vi "GetAllAxisPositions.vi"(8 "error in (no error)":errorcluster, 11 "Picomoto8742ControllerClass in":refnum<class "Picomoto8742ControllerClass.lvclass">) -> (0 "error out":errorcluster, 2 "AxisPositions":i32[](array[numeric]), 3 "Picomoto8742ControllerClass out":refnum<class "Picomoto8742ControllerClass.lvclass">)   [LabVIEW 2020, in "Picomoto8742ControllerClass.lvclass"]
doc: "Query all the axis positions from the physical device"
uses:
  Picomoto8742ControllerClass.lvclass
  Picomoto8742ControllerClass.lvclass/Picomoto8742ControllerClass.ctl
  PicoMotor8742Axis/Picomotor8742Axis.lvclass
panel:
  in  "milliseconds to wait":u32
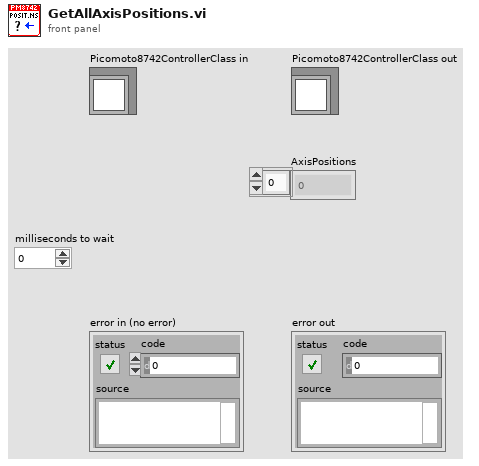
[diagram p1: front panel]
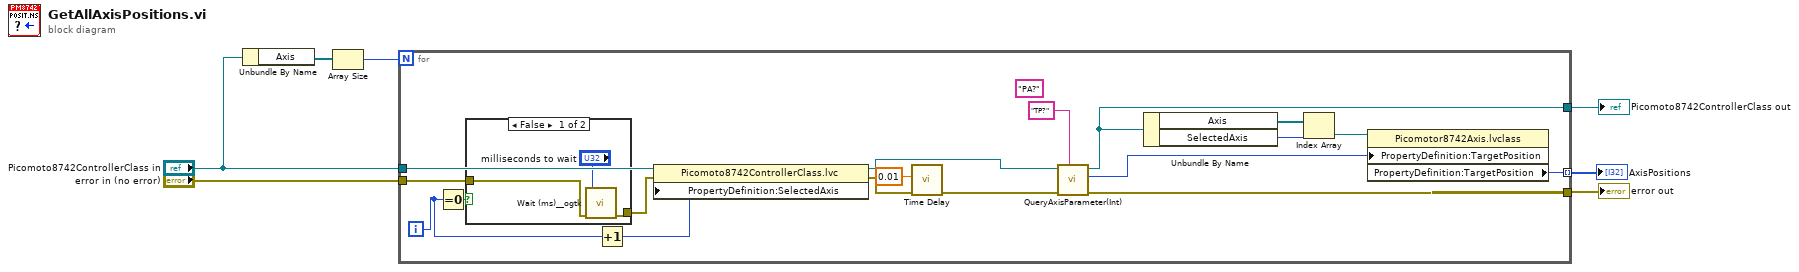
[diagram p0: block diagram]
diagram:
  n1 = Unbundle By Name("Picomoto8742ControllerClass in") -> ("Axis"=w4:refnum<class "Picomotor8742Axis.lvclass">[])
  n2 = Array Size(array=w4) -> (size(s)=w3:i32)
  n3 = for {
    N: w3 -> [_]
    tunnel: "Picomoto8742ControllerClass in" -> [w25]
    tunnel: [w19] -> w6
    tunnel: "error in (no error)" -> [w9]
    tunnel: [w14] -> w1 mode=indexing
    tunnel: [w13] -> w2
    i -> [w11]
    (unwired) "PA?" ("string")
    n4 = Equal To 0?(x=w11) -> (x = 0?=w10:bool)
    n5 = case shown="False" w10 {
      tunnel: w9 -> [w28 w29]
      tunnel: [w27 w29] -> w8
      frame False {
        n6 = call <userlib>:"Wait (ms)__ogtk.vi"("error in (no error)"=w28, "milliseconds to wait"="milliseconds to wait") -> ("error out"=w27:errorcluster)  [unwired: 8 in, 1 out]
      }
      frame True {
      }
    }
    n7 = Increment(x=w11) -> (x+1=w24:i32)
    n8 = property class="Picomoto8742ControllerClass.lvc"(reference=w25, error in=w8, "PropertyDefinition:SelectedAxis"=w24) -> (reference out=w22:refnum<class "Picomoto8742ControllerClass.lvclass">, error out=w21:errorcluster)
    n9 = call "Time Delay"("error in (no error)"=w21, "Delay Time (s)"=0.01) -> ("error out"=w20:errorcluster)  [unwired: 9 in]
    n10 = call-dynamic "QueryAxisParameter(Int).vi"("Cmd"="TP?" ("string"), "error in (no error)"=w20, "Picomoto8742ControllerClass in"=w22) -> ("error out"=w19:errorcluster, "ValueOut"=w15:i32, "Picomoto8742ControllerClass Out"=w13:refnum<class "Picomoto8742ControllerClass.lvclass">)  [unwired: 6 in]
    n11 = Unbundle By Name(w13) -> ("Axis"=w18:refnum<class "Picomotor8742Axis.lvclass">[], "SelectedAxis"=w17:u32)
    n12 = Index Array(array=w18, index=w17) -> (element=w16:refnum<class "Picomotor8742Axis.lvclass">)
    n13 = property class="Picomotor8742Axis.lvclass"(reference=w16, "PropertyDefinition:TargetPosition"=w15) -> ("PropertyDefinition:TargetPosition"=w14:i32)  [unwired: 1 in, 2 out]
  }
  "error out" <- w6
  "Picomoto8742ControllerClass out" <- w2
  "AxisPositions" <- w1
